vi "Actor Core.vi"(8 "error in":errorcluster, 11 "Acquisition in":refnum<class "Acquisition.lvclass">) -> (0 "error out":errorcluster, 3 "Actor out":refnum<class "Actor.lvclass">)   [LabVIEW 2020, in "Acquisition.lvlib" / "Acquisition.lvclass"]
doc: "(<B>Filename</B>: Actor Framework.lvlib:Actor.lvclass:Actor Core.vi)\n\nReceives messages to the actor, reacts to them, and initiates any error handling that may shut the actor down.\n\nDescendant classes may override this VI to append parallel tasks for the actor to complete while it handles messages. Overrides use the Call Parent Class Method node."
uses:
  Acquisition.lvclass
  C:/Program Files (x86)/National Instruments/LabVIEW 2020/vi.lib/ActorFramework/Actor/Actor.lvclass
  <vilib>/ActorFramework/Actor/Actor.lvclass
  <vilib>/ActorFramework/Actor/Actor.lvclass/Actor.ctl
  Acquisition.lvclass/Acquisition.ctl
  Businness Logic/Businness Logic Messages/Data Aquired Msg/Data Aquired Msg.lvclass/Data Aquired Msg.ctl
  <vilib>/ActorFramework/Message Enqueuer/Message Enqueuer.lvclass/Message Enqueuer.ctl
  <vilib>/ActorFramework/Message Enqueuer/Enqueue.vi
  Businness Logic/Businness Logic Messages/Data Aquired Msg/Data Aquired Msg.lvclass
  C:/Program Files (x86)/National Instruments/LabVIEW 2020/vi.lib/ActorFramework/Message/Message.lvclass
  <vilib>/ActorFramework/Message Priority Queue/Priority Enqueue.vi
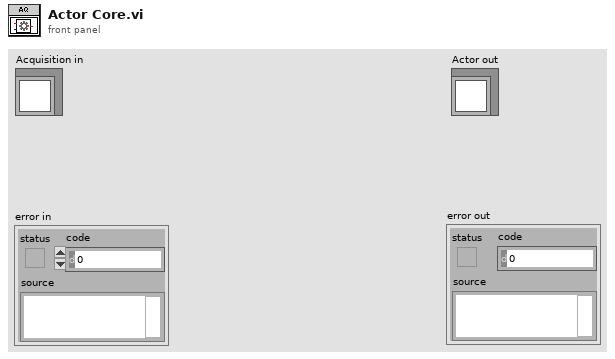
[diagram p1: front panel]
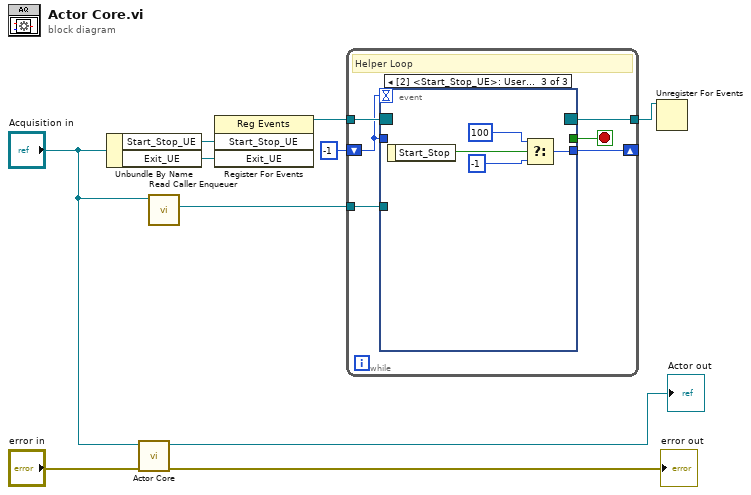
[diagram p0: block diagram]
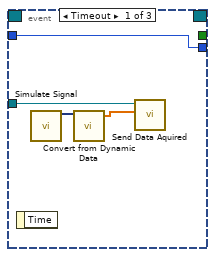
[diagram p2: hidden frame]
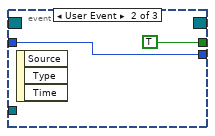
[diagram p3: hidden frame]
diagram:
  n1 = Unbundle By Name("Acquisition in") -> ("Start_Stop_UE"=w5:refnum<user-event>, "Exit_UE"=w4:refnum<user-event>)
  n2 = call-parent "Actor Core.vi"("error in"="error in", "Actor in"="Acquisition in") -> ("error out"=→"error out":errorcluster, "Actor out"=→"Actor out":refnum<class "Actor.lvclass">)  [unwired: 8 in]
  n3 = call <vilib>:"Read Caller Enqueuer.vi"("Actor"="Acquisition in") -> ("Caller Enqueuer"=w1:refnum<class "Message Enqueuer.lvclass">)  [unwired: 10 in]
  n4 = register-events(w5, w4) -> (reference out=w7:refnum<event-registration>)  [unwired: 2 in, 1 out]
  n5 = while {
    tunnel: w7 -> [w16]
    tunnel: [w15] -> w6
    shift-right: [w13] -> _
    shift-left: -1 -> [w12]
    tunnel: w1 -> [w11]
    stop <- w14 stop-if-true
    # "Helper Loop"
    n6 = event shown="[2] <Start_Stop_UE>: User Event" {
      selector: w16 -> [_ _ _]
      dyn-events: [_ _ _] -> w15
      timeout: w12 -> [_ _ _]
      tunnel: [_ TRUE _] -> w14
      tunnel: [w20 w21 w24] -> w13
      tunnel: w12 -> [w20 w21 _]
      tunnel: w11 -> [w17 _ _]
      event Timeout {
        n7 = event-data() -> ()  [unwired: 1 in, 1 out]
        n8 = call "Simulate Signal"() -> ("Sine with Uniform Noise"=w19:dynamicdata)  [unwired: 14 in, 1 out]
        n9 = call "Convert from Dynamic Data"("Dynamic Data Type"=w19) -> ("Array"=w18:dbl[])  [unwired: 3 in]
        n10 = call "Send Data Aquired.vi"("Data"=w18, "Message Enqueuer"=w17) -> ()  [unwired: 8 in, 2 out]
      }
      event User Event {
        n11 = event-data() -> ()  [unwired: 1 in, 3 out]
      }
      event User Event {
        n12 = event-data() -> ("Start_Stop"=w26:bool)  [unwired: 1 in]
        n13 = Select(t=100, s=w26, f=-1) -> (s? t:f=w24:i32)
      }
    }
  }
  n14 = Unregister For Events(event registration refnum=w6) -> ()  [unwired: 1 in, 1 out]
